vi "Read Root.vi"(11 "Setup in":refnum<class "Setup.lvclass">) -> (2 "Root":bool)   [LabVIEW 2025, in "jettl.lvlib" / "Setup.lvlib" / "Setup.lvclass"]
uses:
  Setup.lvclass
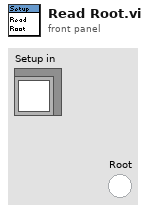
[diagram p1: front panel]
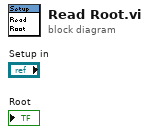
[diagram p0: block diagram]
diagram:
